vi "LVClass_HasoData ctor.vi"(0 "HasoData in":refnum<class "HasoData.lvclass">, 5 "HasoSlopes.lvclass":refnum<class "HasoSlopes.lvclass">, 11 "error in (no error)":errorcluster) -> (4 "HasoData out":refnum<class "HasoData.lvclass">, 15 "error out":errorcluster)   [LabVIEW 2020, in "HasoData.lvclass"]
doc: "HasoData constructor from HasoSlopes.\n\n--------------------------------------------------------------------------------\n\n<B>HasoDataIn </B> : Constant Pointer to HasoData object.\n<B>HasoDataOut </B> : Constant Pointer to HasoData object.\n<B>HasoSlopes </B> : HasoSlopes object.\n<B>ErrorIn </B> : Error\n<B>ErrorOut </B> : Error\n\n--------------------------------------------------------------------------------"
uses:
  HasoData.lvclass
  HasoSlopes.lvclass
  Handle creation.ctl
  HasoData.lvclass/HasoData.ctl
  LVClass_HasoSlopes Read HasoSlopes _ property.vi
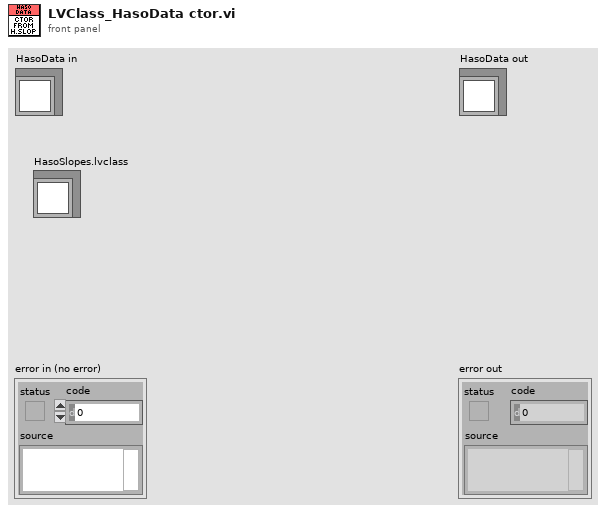
[diagram p1: front panel]
types:
  T1 = typedef "Handle creation.ctl" = enum16{"By ctor", "By write function"}
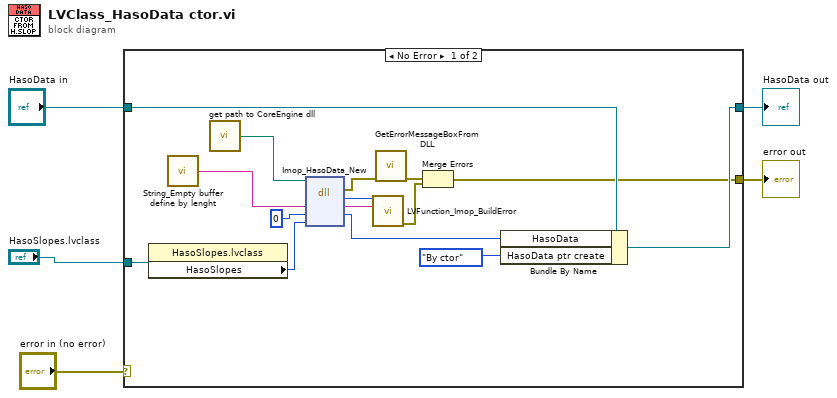
[diagram p0: block diagram]
diagram:
  n1 = case shown="No Error" "error in (no error)" {
    selector: "error in (no error)" -> [_ w22]
    tunnel: [w6 w22] -> w3
    tunnel: [w14 w21] -> w2
    tunnel: "HasoData in" -> [w15 w21]
    tunnel: "HasoSlopes.lvclass" -> [w10 _]
    frame No Error {
      n2 = property class="HasoSlopes.lvclass"(reference=w10) -> ("HasoSlopes"=w9:i32)  [unwired: 1 in, 2 out]
      n3 = call "String_Empty buffer define by lenght.vi"() -> ("Empty buffer"=w16:string)  [unwired: 1 in]
      n4 = call "get path to CoreEngine dll.vi"() -> ("path to c_interface_vc100.dll"=w13:path)  [unwired: 12 in, 3 out]
      n5 = dll-call lib="D:/soft/HASO_v3/SVN_trunk/ImOpCoreEngine4_LV2011/DLLs/c_interface_vc100.dll" fn="Imop_HasoData_New"(path in=w13, "message"=w16, "objet"=0, "haso slopes"=w9) -> (error out=w12:errorcluster, "return type"=w19:i32, "message"=w18:string, "objet"=w17:i32)  [unwired: 3 in, 1 out]
      n6 = call "LVFunction_Imop_BuildError.vi"("code"=w19, "String to Prepend to source (\"\")"=w18) -> ("error out"=w7:errorcluster)  [unwired: 13 in]
      n7 = call "GetErrorMessageBoxFromDLL.vi"("error IN"=w12) -> ("error OUT"=w8:errorcluster)  [unwired: 10 in]
      n8 = Merge Errors(w8, w7) -> (w6:errorcluster)
      n9 = Bundle By Name(cluster=w15, "HasoData"=w17, "HasoData ptr create"=Handle_creation."By ctor") -> (w14:refnum<class "HasoData.lvclass">)
    }
    frame Error {
    }
  }
  "error out" <- w3
  "HasoData out" <- w2
